vi "CreateQueues.vi"(0 "object in":refnum<class "Application.lvclass">, 5 "error in (no error)":errorcluster) -> (14 "object out":refnum<class "Application.lvclass">, 19 "error out":errorcluster)   [LabVIEW 2019, in "Application.lvclass"]
uses:
  Application.lvclass
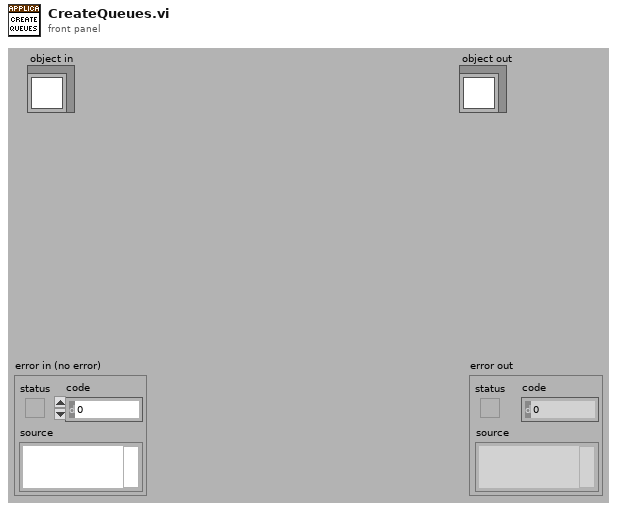
[diagram p1: front panel]
types:
  T1 = cluster{"Message":string, "Message Data":variant}
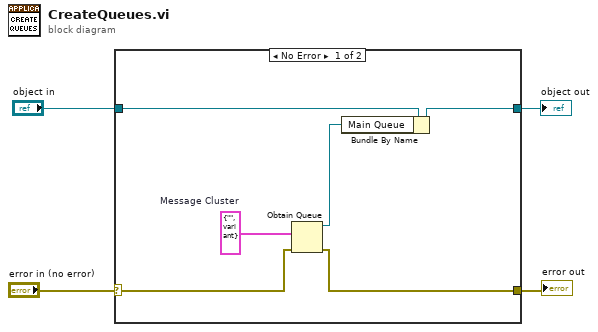
[diagram p0: block diagram]
diagram:
  n1 = case shown="No Error" "error in (no error)" {
    selector: "error in (no error)" -> [w7 w12]
    tunnel: [w6 w12] -> w3
    tunnel: [w8 w11] -> w1
    tunnel: "object in" -> [w10 w11]
    frame No Error {
      w9 = T1 {"Message"="", "Message Data"=variant}  # Message Cluster
      n2 = Obtain Queue(element data type=w9, error in (no error)=w7) -> (queue out=w5:refnum<queue>, error out=w6:errorcluster)  [unwired: 3 in, 1 out]
      n3 = Bundle By Name(cluster=w10, "Main Queue"=w5) -> (w8:refnum<class "Application.lvclass">)
    }
    frame Error {
    }
  }
  "error out" <- w3
  "object out" <- w1
